vi "Obtain Queue and Notifier.vi"(8 "error in (no error)":errorcluster, 11 "Instrument.DAQ in":refnum<class "Instrument.DAQ.lvclass">) -> (0 "error out":errorcluster, 2 "Queue and Notifier":T1, 3 "Instrument.DAQ":refnum<class "Instrument.DAQ.lvclass">)   [LabVIEW 2019, in "Instrument.Lockin.lvlib" / "Instrument.DAQ.lvclass"]
uses:
  Instrument.DAQ.lvclass
  Typedefs/Queue and Notifier.ctl
  C:/Program Files/National Instruments/LabVIEW 2019/vi.lib/JKI/JKI SMO/SMO/SMO.lvclass
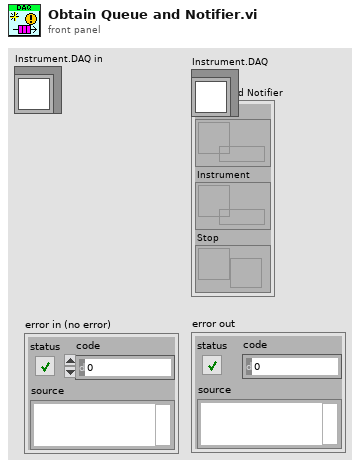
[diagram p1: front panel]
types:
  T1 = typedef "Instrument.Lockin.lvlib/Instrument.DAQ.lvclass/Queue and Notifier.ctl" = cluster{"Message":refnum<queue>, "Instrument":refnum<queue>, "Stop":refnum<notifier>}
  T2 = cluster{"queue out":refnum<queue>, "queue out":refnum<queue>, "notifier out":refnum<notifier>}
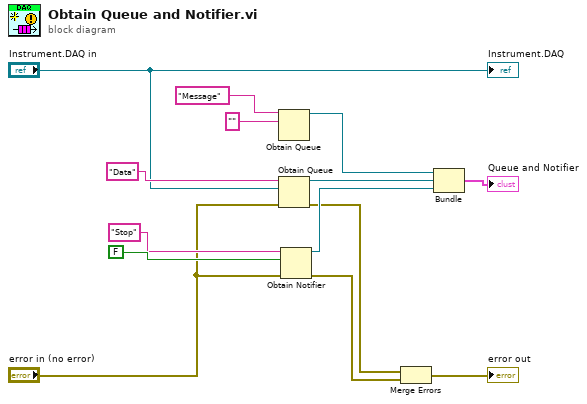
[diagram p0: block diagram]
diagram:
  n1 = Obtain Queue(name (unnamed)="Message", element data type="" ("name (unnamed)")) -> (queue out=w1:refnum<queue>)  [unwired: 3 in, 2 out]
  n2 = Obtain Queue(name (unnamed)="Data", element data type="Instrument.DAQ in", error in (no error)="error in (no error)") -> (queue out=w12:refnum<queue>, error out=w6:errorcluster)  [unwired: 2 in, 1 out]
  n3 = Obtain Notifier(name (unnamed)="Stop", notification data type=FALSE, error in (no error)="error in (no error)") -> (notifier out=w13:refnum<notifier>, error out=w5:errorcluster)  [unwired: 1 in, 1 out]
  n4 = Merge Errors(w6, w5) -> (→"error out":errorcluster)
  n5 = Bundle("queue out"=w1, "queue out"=w12, "notifier out"=w13) -> (→"Queue and Notifier":T2)  [unwired: 1 in]
  "Instrument.DAQ" <- "Instrument.DAQ in"
